vi "CFG_load.vi"(8 "error in":errorcluster, 11 "config file":path) -> (0 "error out":errorcluster, 2 "default folder":path, 3 "config file dup":path)   [LabVIEW 2014]
uses:
  <vilib>/Utility/config.llb/NI_LVConfig.lvlib
  <vilib>/Utility/config.llb/Read Key (Path).vi
  <vilib>/Utility/sysdir.llb/System Directory Type.ctl
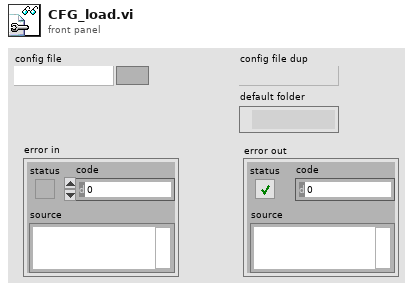
[diagram p1: front panel]
types:
  T1 = typedef "System Directory Type.ctl" = i32
  T2 = typedef "NI_LVConfig.lvlib/Config Data RefNum.ctl" = refnum<k1>
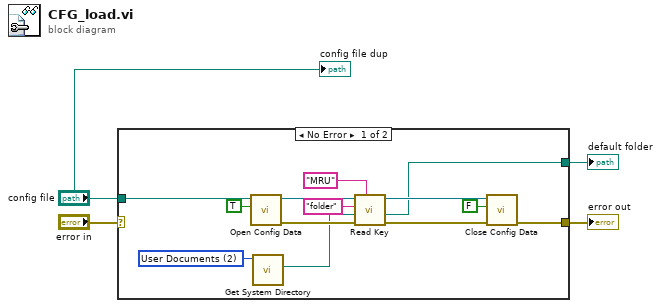
[diagram p0: block diagram]
diagram:
  n1 = case shown="No Error" "error in" {
    tunnel: [w17 _] -> w4
    tunnel: [w9 _] -> w3
    tunnel: "config file" -> [w8 _]
    frame No Error {
      w7 = T1 2 items=["User Home"=0, "User Desktop"=1, "User Documents"=2, "User Application Data"=3, "User Preferences"=4, "User Temporary"=5, "Public Documents"=6, "Public Application Data"=7, "Public Preferences"=8, "Public Cache"=13, "System Core Libraries"=9, "System Installed Libraries"=10, "Application Files"=11, "Boot Volume Root"=12] ("system directory type")
      n2 = call <vilib>:"Open Config Data.vi"("create file if necessary (T)"=TRUE, "configuration file path"=w8) -> ("error out"=w12:errorcluster, "refnum"=w10:T2)  [unwired: 7 in, 1 out]
      n3 = call <vilib>:"Get System Directory.vi"("system directory type"=w7) -> ("system directory"=w6:path)  [unwired: 10 in]
      n4 = call-poly <vilib>:"Read Key.vi"("section"="MRU", "error in (no error)"=w12, "default value"=w6, "key"="folder", "refnum"=w10) -> ("error out"=w13:errorcluster, "value"=w9:path, "refnum out"=w11:T2)  [unwired: 3 in, 1 out]
      n5 = call <vilib>:"Close Config Data.vi"("error in (no error)"=w13, "write file if changed (T)"=FALSE, "refnum"=w11) -> ("error out"=w17:errorcluster)  [unwired: 7 in, 1 out]
    }
    frame Error {
    }
  }
  "error out" <- w4
  "default folder" <- w3
  "config file dup" <- "config file"
